vi "Update Step.vi"(0 "reference in":refnum<class "Recipe.lvclass">, 5 "Index":i32, 7 "Fire (%)":dbl, 9 "Duration (s)":dbl, 11 "Error In":errorcluster) -> (4 "reference out":refnum<class "Recipe.lvclass">, 15 "Error Out":errorcluster)   [LabVIEW 2021, in "Recipe.lvclass"]
uses:
  Recipe.lvclass
  Recipe Step/Recipe Step.lvclass
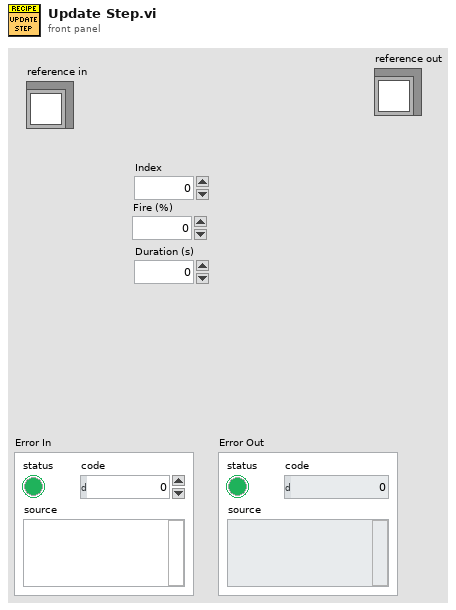
[diagram p1: front panel]
types:
  T1 = typedef "Recipe.lvclass/ObjectAttributes.ctl" = cluster{"Steps":refnum<class "Recipe Step.lvclass">[], "Current Info":cluster{"Current Index":u64}}
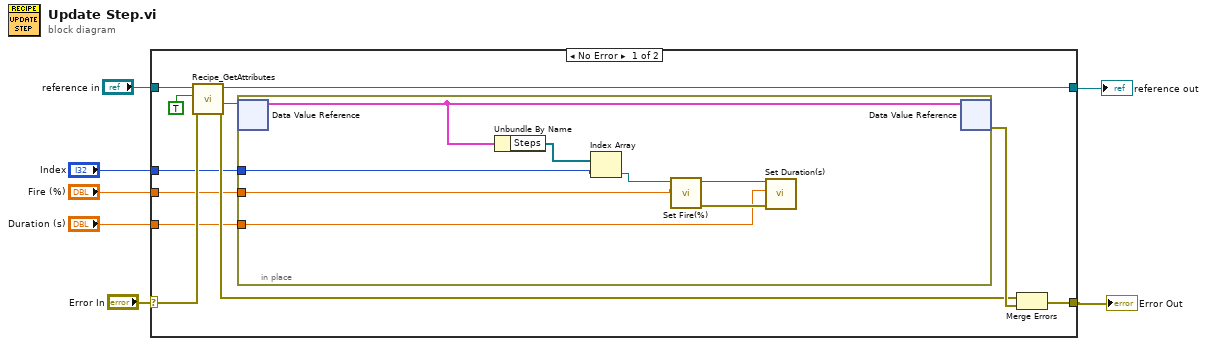
[diagram p0: block diagram]
diagram:
  n1 = case shown="No Error" "Error In" {
    selector: "Error In" -> [w17 w28]
    tunnel: [w14 w28] -> w6
    tunnel: [w15 w27] -> w4
    tunnel: "reference in" -> [w18 w27]
    tunnel: "Index" -> [w10 _]
    tunnel: "Fire (%)" -> [w9 _]
    tunnel: "Duration (s)" -> [w8 _]
    frame No Error {
      n2 = call "Recipe_GetAttributes.vi"("Error In"=w17, "OnlyGetDvrReference(False)"=TRUE, "reference in"=w18) -> ("Error Out"=w12:errorcluster, "DataRef"=w13:refnum<data-value>, "reference out"=w15:refnum<class "Recipe.lvclass">)  [unwired: 5 in, 1 out]
      n3 = in-place {
        in-place-border: w10 -> [w24]
        in-place-border: w9 -> [w20]
        in-place-border: w8 -> [w19]
        n4 = in-place-dvr #1(w13) -> (w26:T1)  [unwired: 1 out]
        n5 = Unbundle By Name(w26) -> ("Steps"=w25:refnum<class "Recipe Step.lvclass">[])
        n6 = Index Array(array=w25, index=w24) -> (element=w23:refnum<class "Recipe Step.lvclass">)
        n7 = call-dynamic "Set Fire(%).vi"("Fire (%)"=w20, "reference in"=w23) -> ("Error Out"=w22:errorcluster, "reference out"=w21:refnum<class "Recipe Step.lvclass">)  [unwired: 8 in]
        n8 = call-dynamic "Set Duration(s).vi"("Error In"=w22, "Duration (s)"=w19, "reference in"=w21) -> ()  [unwired: 7 in, 2 out]
        n9 = in-place-dvr #1(w26) -> (w16:errorcluster)  [unwired: 1 out]
      }
      n10 = Merge Errors(w12, w16) -> (w14:errorcluster)
    }
    frame Error {
    }
  }
  "Error Out" <- w6
  "reference out" <- w4
